vi "Write Digital Lines Wrapper.vi"(0 "Task map in":map{string, refnum<k21>}(c390), 5 "Message Data in":T2, 11 "error in (no error)":errorcluster) -> (4 "Task map out":map{string, refnum<k21>}(c390), 6 "Message Data out":T1, 15 "error out":errorcluster)   [LabVIEW 2021, in "NI DAQmx_wrapper.lvlib"]
uses:
  NI DAQmx_wrapper.lvlib
  NI DAQmx_server/RPC Messages/nidaqmx_grpc_WriteDigitalLinesRequest.ctl
  NI DAQmx_server/RPC Messages/nidevice_grpc_Session_session/nidevice_grpc_Session_session.lvclass
  NI DAQmx_server/RPC Messages/nidaqmx_grpc_WriteDigitalLinesRequest_data_layout_enum/nidaqmx_grpc_WriteDigitalLinesRequest_data_layout_enum.lvclass
  NI DAQmx_server/RPC Messages/nidevice_grpc_Session.ctl
  NI DAQmx_server/RPC Messages/nidaqmx_grpc_WriteDigitalLinesResponse.ctl
  NI DAQmx_server/RPC Messages/nidevice_grpc_Session_session/nidevice_grpc_Session_session.lvclass/nidevice_grpc_Session_session.ctl
  <vilib>/DAQmx/write.llb/DAQmx Write (Digital Bool 1Line 1Point).vi
  <vilib>/DAQmx/miscellaneous.llb/DAQmx Fill In Error Info.vi
  NI DAQmx_server/NI DAQmx_server.lvlib
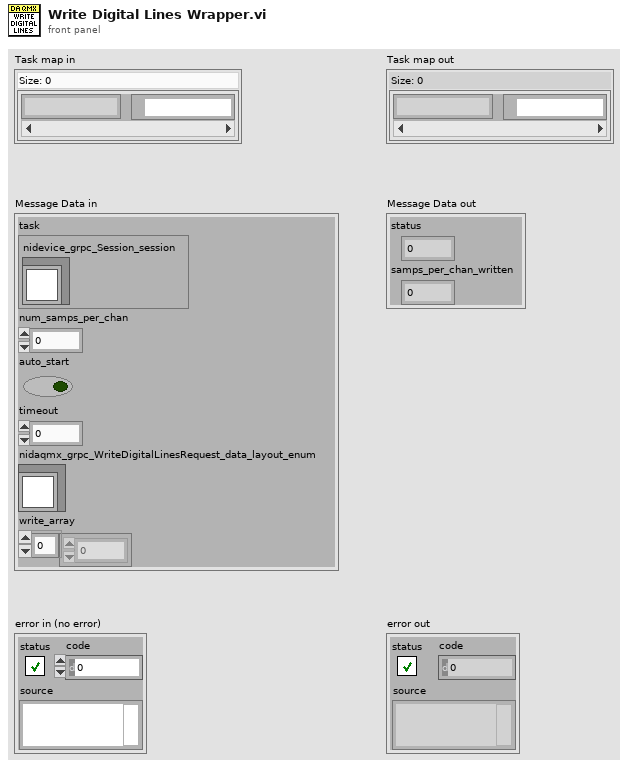
[diagram p1: front panel]
types:
  T1 = typedef "NI DAQmx_server.lvlib/nidaqmx_grpc_WriteDigitalLinesResponse.ctl" = cluster{"status":i32, "samps_per_chan_written":i32}
  T2 = typedef "NI DAQmx_server.lvlib/nidaqmx_grpc_WriteDigitalLinesRequest.ctl" = cluster{"task":T3, "num_samps_per_chan":i32, "auto_start":bool, "timeout":dbl, "nidaqmx_grpc_WriteDigitalLinesRequest_data_layout_enum":refnum<class "nidaqmx_grpc_WriteDigitalLinesRequest_data_layout_enum.lvclass">, "write_array":u8[]}
  T3 = typedef "NI DAQmx_server.lvlib/nidevice_grpc_Session.ctl" = cluster{"nidevice_grpc_Session_session":refnum<class "nidevice_grpc_Session_session.lvclass">}
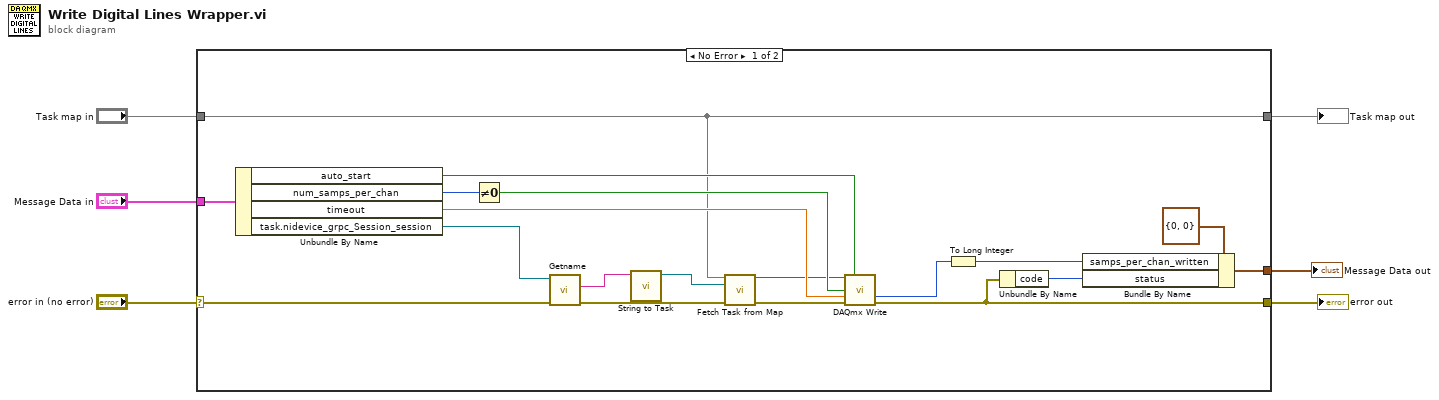
[diagram p0: block diagram]
diagram:
  n1 = case shown="No Error" "error in (no error)" {
    selector: "error in (no error)" -> [w14 w27]
    tunnel: [w23 w27] -> w5
    tunnel: "Task map in" -> [w7 w26]
    tunnel: [w7 w26] -> w3
    tunnel: "Message Data in" -> [w25 _]
    tunnel: [w8 _] -> w1
    frame No Error {
      n2 = Unbundle By Name(w25) -> ("auto_start"=w22:bool, "num_samps_per_chan"=w18:i32, "timeout"=w21:dbl, "task.nidevice_grpc_Session_session"=w12:refnum<class "nidevice_grpc_Session_session.lvclass">)
      n3 = Not Equal To 0?(x=w18) -> (x != 0?=w19:bool)
      n4 = call "Getname.vi"("error in (no error)"=w14, "OneOfTemplate in"=w12) -> ("error out"=w16:errorcluster, "Get_Val"=w17:string)  [unwired: 7 in, 1 out]
      n5 = call "String to Task.vi"("Get_Val"=w17) -> ("Refnum out"=w15:refnum<k21>)  [unwired: 10 in]
      n6 = call "Fetch Task from Map.vi"("Task map in"=w7, "Task in"=w15, "error in (no error)"=w16) -> ("Task out"=w11:refnum<k21>, "error out"=w13:errorcluster)  [unwired: 10 in, 1 out]
      n7 = call-poly <vilib>:"DAQmx Write.vi"("task/channels in"=w11, "auto start"=w22, "data"=w19, "timeout"=w21, "error in"=w13) -> ("number of samples written per channel"=w10:u32, "error out"=w23:errorcluster)  [unwired: 8 in, 1 out]
      n8 = To Long Integer(number=w10) -> (32bit integer=w9:i32)
      n9 = Unbundle By Name(w23) -> ("code"=w24:i32)
      n10 = Bundle By Name(cluster=T1 {"status"=0, "samps_per_chan_written"=0} ("Message Data"), "samps_per_chan_written"=w9, "status"=w24) -> (w8:T1)
    }
    frame Error {
    }
  }
  "error out" <- w5
  "Task map out" <- w3
  "Message Data out" <- w1
